vi "Compute_Layer_Id_Patch_Permutationsvi.vi"(7 "Limit":u16, 10 "Patch Sizes":i32[](array[numeric]), 11 "Layer IDs":i32[](array[numeric])) -> (3 "LayerID,PatchSize Permutations":T1[](array[typedef]))   [LabVIEW 2024]
uses:
  <vilib>/Ngene/DeepLTK Anomaly Detection Addon/DeepLTK_Anomaly_Detection_Addon/API/Controls/Feature_Layer_Selector.ctl
  <vilib>/Ngene/DeepLTK Anomaly Detection Addon/DeepLTK_Anomaly_Detection_Addon/DeepLTK_Anomaly_Detection_Addon.lvlib
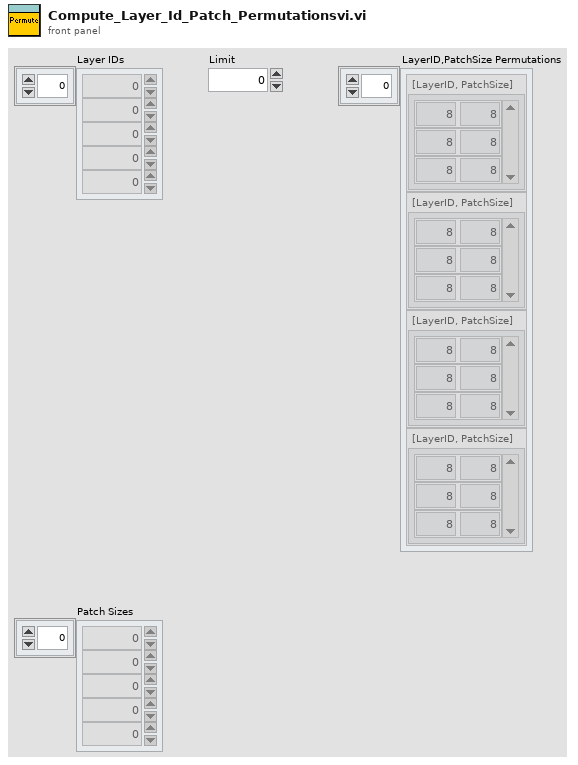
[diagram p1: front panel]
types:
  T1 = typedef "DeepLTK_Anomaly_Detection_Addon.lvlib/Feature_Layer_Selector.ctl" = cluster{"[LayerID, PatchSize]":cluster{"Layer_ID":i32, "Patch_Size":i32}[]}
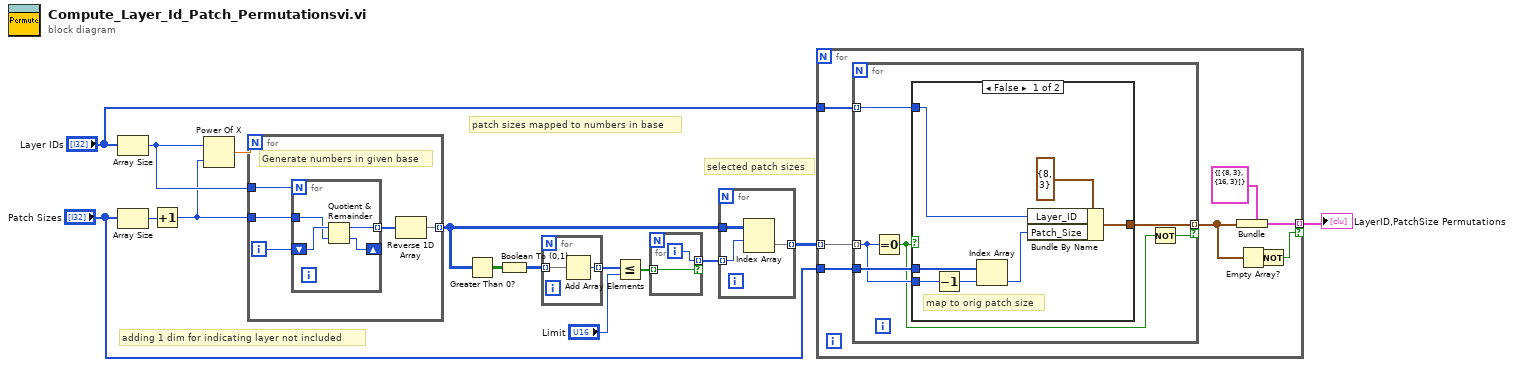
[diagram p0: block diagram]
diagram:
  # "patch sizes mapped to numbers in base"
  # "adding 1 dim for indicating layer not included"
  # "selected patch sizes"
  n1 = Array Size(array="Layer IDs") -> (size(s)=w13:i32)
  n2 = Array Size(array="Patch Sizes") -> (size(s)=w15:i32)
  n3 = Increment(x=w15) -> (x+1=w12:i32)
  n4 = Power Of X(1:w12, 2:w13) -> (0:w14:dbl)
  n5 = for {
    N: w14 -> [_]
    tunnel: w13 -> [w19]
    tunnel: [w17] -> w6 mode=indexing
    tunnel: w12 -> [w16]
    i -> [w20]
    # "Generate numbers in given base"
    n6 = for {
      N: w19 -> [_]
      tunnel: w16 -> [w23]
      tunnel: [w22] -> w18 mode=indexing
      shift-right: [w21] -> _
      shift-left: w20 -> [w24]
      n7 = Quotient & Remainder(x=w24, y=w23) -> (x-y*floor(x/y)=w22:i32, floor(x/y)=w21:i32)
    }
    n8 = Reverse 1D Array(array=w18) -> (reversed array=w17:i32[])
  }
  n9 = Greater Than 0?(x=w6) -> (x > 0?=w11:bool[][])
  n10 = Boolean To (0,1)(Boolean=w11) -> (0, 1=w10:i16[][])
  n11 = for {
    tunnel: w10 -> [w26] mode=indexing
    tunnel: [w25] -> w9 mode=indexing
    n12 = Add Array Elements(numeric array=w26) -> (sum=w25:i16)
  }
  n13 = Less Or Equal?(x=w9, y="Limit") -> (x <= y?=w7:bool[])
  n14 = for {
    tunnel: w7 -> [w27] mode=indexing
    tunnel: [w28] -> w5 mode=indexing if=w27
    i -> [w28]
  }
  n15 = for {
    tunnel: w6 -> [w31]
    tunnel: w5 -> [w30] mode=indexing
    tunnel: [w29] -> w4 mode=indexing
    n16 = Index Array(array=w31, index (row)=w30) -> (element=w29:i32[])  [unwired: 1 in]
  }
  n17 = for {
    tunnel: w4 -> [w39] mode=indexing
    tunnel: "Layer IDs" -> [w38]
    tunnel: "Patch Sizes" -> [w37]
    tunnel: [w35] -> w1 mode=indexing if=w32
    n18 = for {
      tunnel: w39 -> [w44] mode=indexing
      tunnel: w38 -> [w43] mode=indexing
      tunnel: w37 -> [w45]
      tunnel: [w42] -> w34 mode=indexing if=w40
      n19 = Equal To 0?(x=w44) -> (x = 0?=w41:bool)
      n20 = case shown="False" w41 {
        tunnel: w45 -> [w52 _]
        tunnel: w44 -> [w51 _]
        tunnel: w43 -> [w49 _]
        tunnel: [w47 _] -> w42
        frame False {
          # "map to orig patch size"
          n21 = Decrement(x=w51) -> (x-1=w46:i32)
          n22 = Index Array(array=w52, index=w46) -> (element=w48:i32)
          n23 = Bundle By Name(cluster=cluster{"Layer_ID":i32, "Patch_Size":i32} {"Layer_ID"=8, "Patch_Size"=3} ("Cluster"), "Layer_ID"=w49, "Patch_Size"=w48) -> (w47:cluster{"Layer_ID":i32, "Patch_Size":i32})
        }
        frame True {
          # "skip"
        }
      }
      n24 = Not(x=w41) -> (.not. x?=w40:bool)
    }
    n25 = Bundle(cluster=T1 {"[LayerID, PatchSize]"=[{"Layer_ID"=8, "Patch_Size"=3}, {"Layer_ID"=16, "Patch_Size"=3}]} ("Feature_Layers 2"), "[LayerID, PatchSize]"=w34) -> (w35:T1)
    n26 = Empty Array?(array=w34) -> (empty?=w33:bool)
    n27 = Not(x=w33) -> (.not. x?=w32:bool)
  }
  "LayerID,PatchSize Permutations" <- w1
